vi "Light Write.vi"(4 "Color":u32(colorbox), 6 "Intensity":u32, 8 "error in (no error)":errorcluster, 9 "Channel":u32, 11 "Lighting Refnum In":refnum<k1>) -> (0 "error out":errorcluster, 3 "Lighting Refnum Out":refnum<k1>)   [LabVIEW 2009]
doc: "Writes the intensity and color information to a particular channel."
uses:
  Refnum Enum.ctl
panel:
  # "Input Data"
  # "Local Data"
  # "Output Data"
  # "No Local Data"
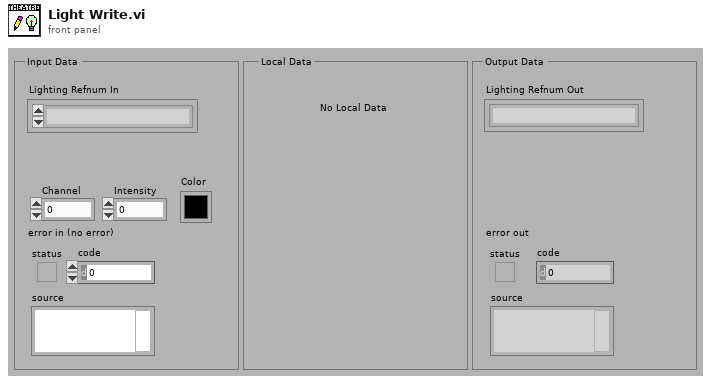
[diagram p1: front panel]
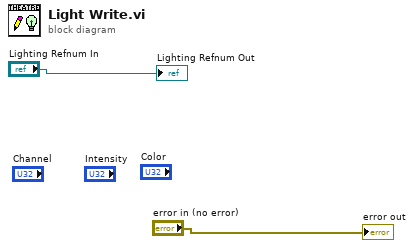
[diagram p0: block diagram]
diagram:
  "error out" <- "error in (no error)"
  "Lighting Refnum Out" <- "Lighting Refnum In"
